vi "Generate Error based LabView error.vi"(4 "Deactive Save Error?":bool, 5 "Actions":T1, 6 "Delete Call Chain?":bool, 7 "Comment":string, 8 "Error In":errorcluster, 9 "Error Classification":T3=enum."LabView built-in", 10 "Source":T4, 11 "ErrorLog Ref":refnum<class "ErrorLog.lvclass">) -> (0 "Error Out":errorcluster, 3 "Error":refnum<class "Error.lvclass">)   [LabVIEW 2019, in "Error.lvclass"]
uses:
  Error.lvclass
  SubModules/ErrorLog/ErrorLog.lvclass
  SubModules/LogsAbstract/TypeDef/Event Source.ctl
  TypeDef/Error Classification.ctl
  EventsAbstract/TypeDef/Event Actions.ctl
  Modules/ModuleAbstract/TypeDef/Module Actions.ctl
  <vilib>/ActorFramework/Message Enqueuer/Message Enqueuer.lvclass
  Error.lvclass/Error.ctl
  Modules/ModuleAbstract/ModuleAbstract.lvclass
  EventsAbstract/EventsAbstract.lvclass
  SubModules/LogsAbstract/LogsAbstract.lvclass
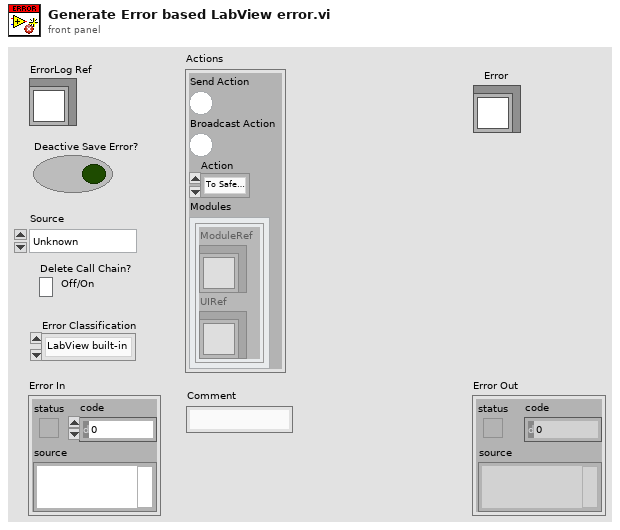
[diagram p1: front panel]
types:
  T1 = typedef "EventsAbstract.lvclass/Event Actions.ctl" = cluster{"Send Action":bool, "Broadcast Action":bool, "Action":T2, "Modules":cluster{"ModuleRef":refnum<class "Message Enqueuer.lvclass">, "UIRef":refnum<class "Message Enqueuer.lvclass">}[]}
  T2 = typedef "ModuleAbstract.lvlib/ModuleAbstract.lvclass/Module Actions.ctl" = enum16{"To Safe State", "Reset Safe State", "Close Module"}
  T3 = typedef "Error.lvclass/Error Classification.ctl" = enum16{"System Error", "Process Error", "Warning", "LabView built-in"}
  T4 = typedef "LogsAbstract.lvlib/LogsAbstract.lvclass/Event Source.ctl" = enum16{"Unknown", "< --- Modules --- >", "Core", "< --- SubModules --- >", "EventLog -> Core", "ErrorLog -> Core"}
  T5 = cluster{"Error?":bool, "Error Code":i32, "Classification":T3, "Call Chain":string}
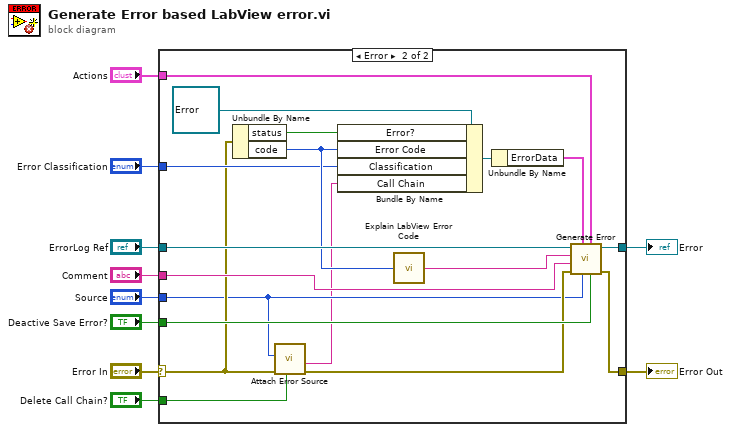
[diagram p0: block diagram]
diagram:
  n1 = case shown="Error" "Error In" {
    selector: "Error In" -> [w11 w16]
    tunnel: [w11 w21] -> w9
    tunnel: [_ w29] -> w8
    tunnel: "Source" -> [_ w14]
    tunnel: "ErrorLog Ref" -> [_ w23]
    tunnel: "Deactive Save Error?" -> [_ w20]
    tunnel: "Error Classification" -> [_ w19]
    tunnel: "Actions" -> [_ w18]
    tunnel: "Comment" -> [_ w17]
    tunnel: "Delete Call Chain?" -> [_ w12]
    frame No Error {
    }
    frame Error {
      n2 = Unbundle By Name(w16) -> ("status"=w27:bool, "code"=w22:i32)
      n3 = call "Attach Error Source.vi"("Delete Call Chain?"=w12, "Error In"=w16, "Error Source"=w14) -> ("Error Out"=w15:errorcluster, "Call Chain"=w13:string)  [unwired: 6 in, 1 out]
      n4 = Bundle By Name(cluster=refnum<class "Error.lvclass"> refnum ("Error.lvclass"), "Error?"=w27, "Error Code"=w22, "Classification"=w19, "Call Chain"=w13) -> (w26:refnum<class "Error.lvclass">)
      n5 = call "Explain LabView Error Code.vi"("Error Code"=w22) -> ("Error Text"=w25:string)
      n6 = Unbundle By Name(w26) -> ("ErrorData"=w24:T5)
      n7 = call "Generate Error.vi"("Deactive Save Error?"=w20, "Actions"=w18, "Source"=w14, "ErrorData"=w24, "Error In"=w15, "Comment"=w17, "Description"=w25, "ErrorLog REF"=w23) -> ("Error Out"=w21:errorcluster, "Error"=w29:refnum<class "Error.lvclass">)  [unwired: 2 in]
    }
  }
  "Error Out" <- w9
  "Error" <- w8
